vi "Read SS2 DAQ Parameters.vi"(8 "error in (no error)":errorcluster, 11 "group in":T3 format="%.0x") -> (0 "error out":errorcluster, 1 "FPGA Parameters":T1 {"gs_psincdec 3" format="%0.0f"; "gs_psincdec 2" format="%0.0f"; "gs_psincdec_1" format="%0.0f"; "gs_no_shift_adj_3" format="%0.0f"; "gs_no_shift_adj_2" format="%0.0f"; "gs_psincdec_0" format="%0.0f"}, 2 "DAQ Parameters":T2 {"# Gate Positions" format="%0.0f"; "Gate Offset" format="%0.0f"; "Bitness" format="%0.0f"; "# Gate Set" format="%0.0f"}, 3 "group out":T3 format="%.0x")   [LabVIEW 2021, in "SwissSPAD.lvlib"]
uses:
  SwissSPAD.lvlib
  <vilib>/addons/h5labview2/base/hid_t.ctl
  SS2 DAQ Parameters.ctl
  SS2 FPGA Parameters.ctl
  SS2 DAQ Parameters List.ctl
  <vilib>/addons/h5labview2/base/lib_path.vi
  <vilib>/addons/h5labview2/base/H5Equery.vi
  <vilib>/addons/h5labview2/dataset/H5Dread.llb/H5Dread.xnode
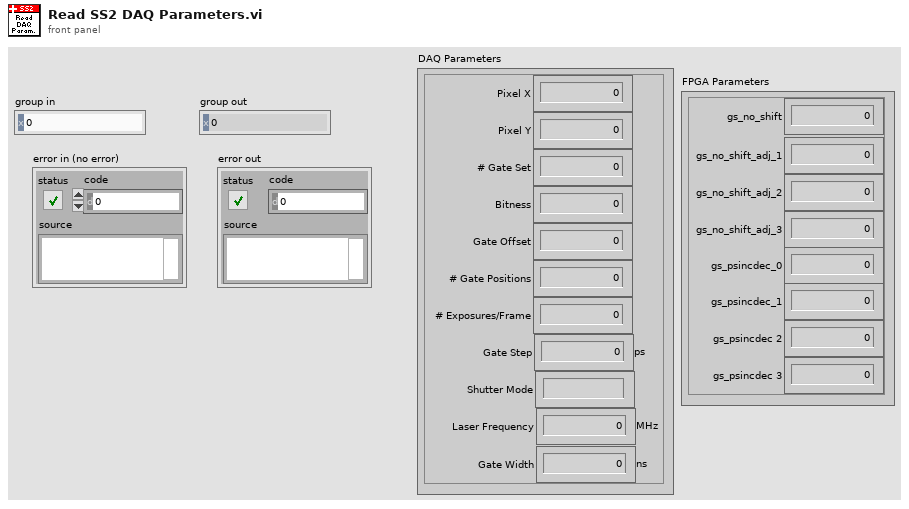
[diagram p1: front panel]
types:
  T1 = typedef "SwissSPAD.lvlib/SS2 FPGA Parameters.ctl" = cluster{"gs_no_shift":i32, "gs_no_shift_adj_1":u32, "gs_no_shift_adj_2":u32, "gs_no_shift_adj_3":u32, "gs_psincdec_0":i32, "gs_psincdec_1":u32, "gs_psincdec 2":u32, "gs_psincdec 3":u32}
  T2 = typedef "SwissSPAD.lvlib/SS2 DAQ Parameters.ctl" = cluster{"Pixel X":i32, "Pixel Y":i32, "# Gate Set":i32, "Bitness":i32, "Gate Offset":i32, "# Gate Positions":i32, "# Exposures/Frame ":i32, "Gate Step":dbl[unit], "Shutter Mode":string, "Laser Frequency":dbl[unit], "Gate Width":dbl[unit]}
  T3 = typedef "hid_t.ctl" = i64
  T4 = typedef "SwissSPAD.lvlib/SS2 DAQ Parameters List.ctl" = enum16{"---DAQ Parameters---", "bits_10", "exp_no_seq", "gate_offset", "gate_set_no", "gate_step_ps", "gs_no_shift", "no_gate_pos", "pixel_x", "pixel_y", "shutter_mode", "gate_width_ns", "laser_f_MHz", "---FPGA Parameters---", "gs_no_shift_adj_1", "gs_no_shift_adj_2", "gs_no_shift_adj_3", "gs_psincdec_0", "gs_psincdec_1", "gs_psincdec_2", "gs_psincdec_3"}
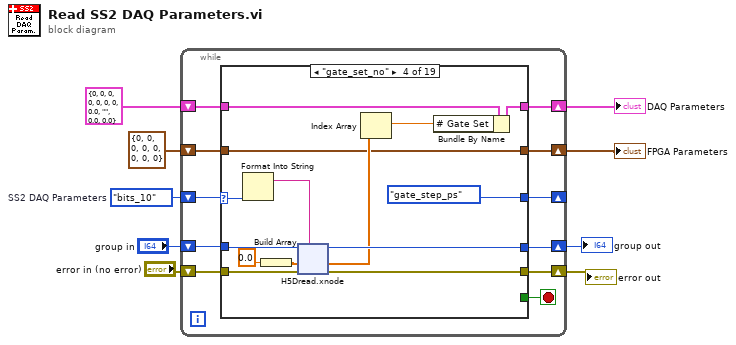
[diagram p0: block diagram]
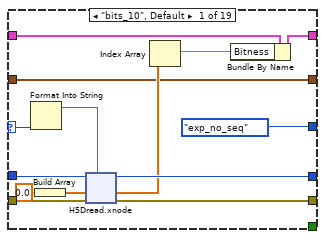
[diagram p2: hidden frame]
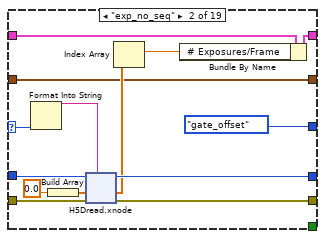
[diagram p3: hidden frame]
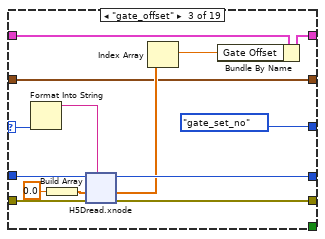
[diagram p4: hidden frame]
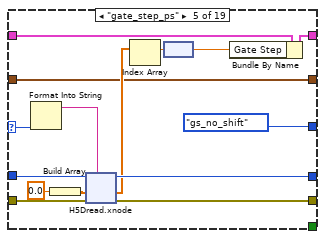
[diagram p5: hidden frame]
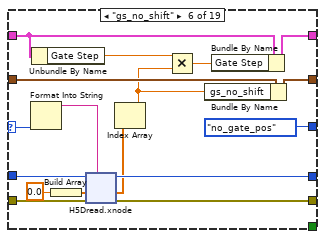
[diagram p6: hidden frame]
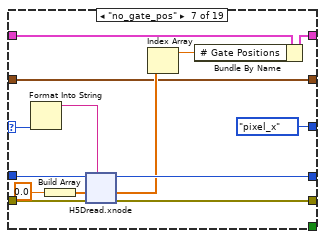
[diagram p7: hidden frame]
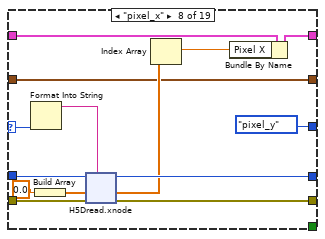
[diagram p8: hidden frame]
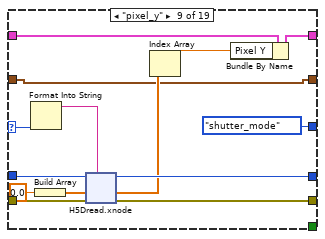
[diagram p9: hidden frame]
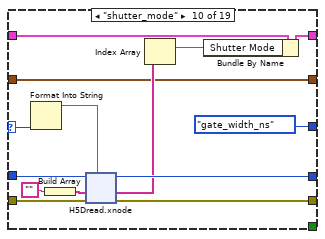
[diagram p10: hidden frame]
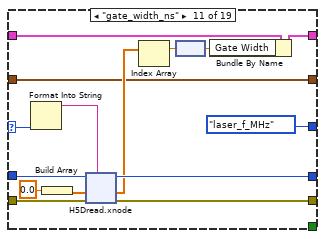
[diagram p11: hidden frame]
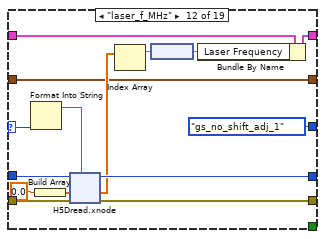
[diagram p12: hidden frame]
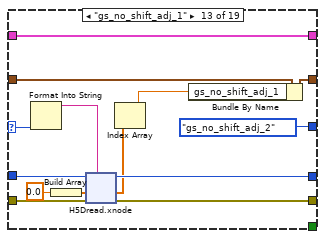
[diagram p13: hidden frame]
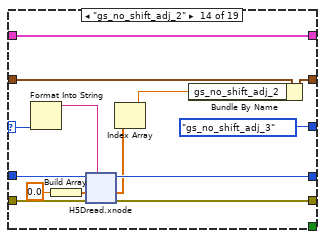
[diagram p14: hidden frame]
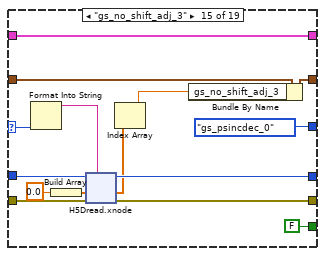
[diagram p15: hidden frame]
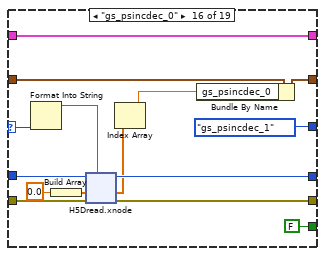
[diagram p16: hidden frame]
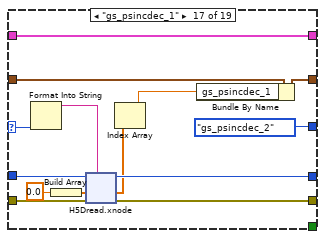
[diagram p17: hidden frame]
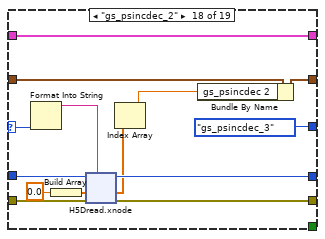
[diagram p18: hidden frame]
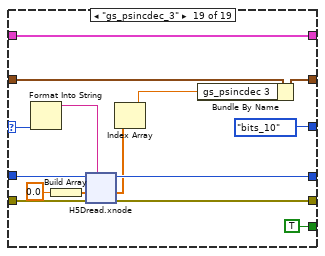
[diagram p19: hidden frame]
diagram:
  w5 = SS2_DAQ_Parameters_List."bits_10"  # SS2 DAQ Parameters
  n1 = while {
    shift-right: [w14] -> w8
    shift-left: T2 {"Pixel X"=0, "Pixel Y"=0, "# Gate Set"=0, "Bitness"=0, "Gate Offset"=0, "# Gate Positions"=0, "# Exposures/Frame "=0, "Gate Step"=0.0, "Shutter Mode"="", "Laser Frequency"=0.0, "Gate Width"=0.0} ("DAQ Parameters") -> [w15]
    shift-right: [w16] -> w6
    shift-left: "error in (no error)" -> [w17]
    shift-right: [w18] -> w3
    shift-left: "group in" -> [w19]
    shift-right: [w12] -> _
    shift-left: w5 -> [w20]
    shift-right: [w10] -> w1
    shift-left: T1 {"gs_no_shift"=0, "gs_no_shift_adj_1"=0, "gs_no_shift_adj_2"=0, "gs_no_shift_adj_3"=0, "gs_psincdec_0"=0, "gs_psincdec_1"=0, "gs_psincdec 2"=0, "gs_psincdec 3"=0} ("FPGA Parameters") -> [w11]
    stop <- w13 stop-if-true
    n2 = case shown="\"gate_set_no\"" w20 {
      selector: w20 -> [w33 w62 w91 w120 w150 w182 w211 w240 w269 w298 w328 w358 w387 w416 w446 w476 w505 w534 w564]
      tunnel: w19 -> [w32 w61 w90 w119 w149 w181 w210 w239 w268 w297 w327 w357 w386 w415 w445 w475 w504 w533 w563]
      tunnel: [w31 w60 w89 w118 w148 w180 w209 w238 w267 w296 w326 w356 w385 w414 w444 w474 w503 w532 w562] -> w18
      tunnel: w17 -> [w30 w59 w88 w117 w147 w179 w208 w237 w266 w295 w325 w355 w384 w413 w443 w473 w502 w531 w561]
      tunnel: [w29 w58 w87 w116 w146 w178 w207 w236 w265 w294 w324 w354 w383 w412 w442 w472 w501 w530 w560] -> w16
      tunnel: w15 -> [w27 w56 w85 w114 w144 w170 w205 w234 w263 w292 w323 w352 w377 w406 w436 w466 w495 w524 w554]
      tunnel: [w25 w54 w83 w112 w142 w171 w203 w232 w261 w290 w321 w350 w377 w406 w436 w466 w495 w524 w554] -> w14
      tunnel: [_ _ _ _ _ _ _ _ _ _ _ _ _ _ FALSE FALSE _ _ TRUE] -> w13
      tunnel: [SS2_DAQ_Parameters_List."exp_no_seq" ("SS2 DAQ Parameters") SS2_DAQ_Parameters_List."gate_offset" ("SS2 DAQ Parameters") SS2_DAQ_Parameters_List."gate_set_no" ("SS2 DAQ Parameters") SS2_DAQ_Parameters_List."gate_step_ps" ("SS2 DAQ Parameters") SS2_DAQ_Parameters_List."gs_no_shift" ("SS2 DAQ Parameters") SS2_DAQ_Parameters_List."no_gate_pos" ("SS2 DAQ Parameters") SS2_DAQ_Parameters_List."pixel_x" ("SS2 DAQ Parameters") SS2_DAQ_Parameters_List."pixel_y" ("SS2 DAQ Parameters") SS2_DAQ_Parameters_List."shutter_mode" ("SS2 DAQ Parameters") SS2_DAQ_Parameters_List."gate_width_ns" ("SS2 DAQ Parameters") SS2_DAQ_Parameters_List."laser_f_MHz" ("SS2 DAQ Parameters") SS2_DAQ_Parameters_List."gs_no_shift_adj_1" ("SS2 DAQ Parameters") SS2_DAQ_Parameters_List."gs_no_shift_adj_2" ("SS2 DAQ Parameters") SS2_DAQ_Parameters_List."gs_no_shift_adj_3" ("SS2 DAQ Parameters") SS2_DAQ_Parameters_List."gs_psincdec_0" ("SS2 DAQ Parameters") SS2_DAQ_Parameters_List."gs_psincdec_1" ("SS2 DAQ Parameters") SS2_DAQ_Parameters_List."gs_psincdec_2" ("SS2 DAQ Parameters") SS2_DAQ_Parameters_List."gs_psincdec_3" ("SS2 DAQ Parameters") SS2_DAQ_Parameters_List."bits_10" ("SS2 DAQ Parameters")] -> w12
      tunnel: w11 -> [w21 w50 w79 w108 w137 w173 w199 w228 w257 w286 w318 w345 w376 w405 w435 w465 w494 w523 w553]
      tunnel: [w21 w50 w79 w108 w137 w172 w199 w228 w257 w286 w318 w345 w375 w404 w434 w464 w493 w522 w552] -> w10
      frame "bits_10", Default {
        n3 = Format Into String(w33) -> (resulting string=w34:string)  [unwired: 3 in, 1 out]
        n4 = Build Array(0.0) -> (w24:dbl[])
        n5 = xnode "H5Dread.xnode"("dataset name (this)"=w34, "error in (no error)"=w30, "default"=w24, "ref in"=w32) -> ("error out"=w29:errorcluster, "data"=w26:dbl[], "ref out"=w31:T3)  [unwired: 2 in, 1 out]
        n6 = Index Array(array=w26) -> (element=w23:dbl)  [unwired: 1 in]
        n7 = Bundle By Name(cluster=w27, "Bitness"=w23) -> (w25:T2)
      }
      frame "exp_no_seq" {
        n8 = Format Into String(w62) -> (resulting string=w63:string)  [unwired: 3 in, 1 out]
        n9 = Build Array(0.0) -> (w53:dbl[])
        n10 = xnode "H5Dread.xnode"("dataset name (this)"=w63, "error in (no error)"=w59, "default"=w53, "ref in"=w61) -> ("error out"=w58:errorcluster, "data"=w55:dbl[], "ref out"=w60:T3)  [unwired: 2 in, 1 out]
        n11 = Index Array(array=w55) -> (element=w52:dbl)  [unwired: 1 in]
        n12 = Bundle By Name(cluster=w56, "# Exposures/Frame"=w52) -> (w54:T2)
      }
      frame "gate_offset" {
        n13 = Format Into String(w91) -> (resulting string=w92:string)  [unwired: 3 in, 1 out]
        n14 = Build Array(0.0) -> (w82:dbl[])
        n15 = xnode "H5Dread.xnode"("dataset name (this)"=w92, "error in (no error)"=w88, "default"=w82, "ref in"=w90) -> ("error out"=w87:errorcluster, "data"=w84:dbl[], "ref out"=w89:T3)  [unwired: 2 in, 1 out]
        n16 = Index Array(array=w84) -> (element=w81:dbl)  [unwired: 1 in]
        n17 = Bundle By Name(cluster=w85, "Gate Offset"=w81) -> (w83:T2)
      }
      frame "gate_set_no" {
        n18 = Format Into String(w120) -> (resulting string=w121:string)  [unwired: 3 in, 1 out]
        n19 = Build Array(0.0) -> (w111:dbl[])
        n20 = xnode "H5Dread.xnode"("dataset name (this)"=w121, "error in (no error)"=w117, "default"=w111, "ref in"=w119) -> ("error out"=w116:errorcluster, "data"=w113:dbl[], "ref out"=w118:T3)  [unwired: 2 in, 1 out]
        n21 = Index Array(array=w113) -> (element=w110:dbl)  [unwired: 1 in]
        n22 = Bundle By Name(cluster=w114, "# Gate Set"=w110) -> (w112:T2)
      }
      frame "gate_step_ps" {
        n23 = Format Into String(w150) -> (resulting string=w151:string)  [unwired: 3 in, 1 out]
        n24 = Build Array(0.0) -> (w141:dbl[])
        n25 = xnode "H5Dread.xnode"("dataset name (this)"=w151, "error in (no error)"=w147, "default"=w141, "ref in"=w149) -> ("error out"=w146:errorcluster, "data"=w143:dbl[], "ref out"=w148:T3)  [unwired: 2 in, 1 out]
        n26 = Index Array(array=w143) -> (element=w140:dbl)  [unwired: 1 in]
        n27 = node(w140) -> (w138:dbl[unit])
        n28 = Bundle By Name(cluster=w144, "Gate Step"=w138) -> (w142:T2)
      }
      frame "gs_no_shift" {
        n29 = Format Into String(w182) -> (resulting string=w183:string)  [unwired: 3 in, 1 out]
        n30 = Unbundle By Name(w170) -> ("Gate Step"=w169:dbl[unit])
        n31 = Build Array(0.0) -> (w175:dbl[])
        n32 = xnode "H5Dread.xnode"("dataset name (this)"=w183, "error in (no error)"=w179, "default"=w175, "ref in"=w181) -> ("error out"=w178:errorcluster, "data"=w176:dbl[], "ref out"=w180:T3)  [unwired: 2 in, 1 out]
        n33 = Index Array(array=w176) -> (element=w168:dbl)  [unwired: 1 in]
        n34 = Multiply(x=w169, y=w168) -> (x*y=w167:dbl[unit])
        n35 = Bundle By Name(cluster=w173, "gs_no_shift"=w168) -> (w172:T1)
        n36 = Bundle By Name(cluster=w170, "Gate Step"=w167) -> (w171:T2)
      }
      frame "no_gate_pos" {
        n37 = Format Into String(w211) -> (resulting string=w212:string)  [unwired: 3 in, 1 out]
        n38 = Build Array(0.0) -> (w202:dbl[])
        n39 = xnode "H5Dread.xnode"("dataset name (this)"=w212, "error in (no error)"=w208, "default"=w202, "ref in"=w210) -> ("error out"=w207:errorcluster, "data"=w204:dbl[], "ref out"=w209:T3)  [unwired: 2 in, 1 out]
        n40 = Index Array(array=w204) -> (element=w201:dbl)  [unwired: 1 in]
        n41 = Bundle By Name(cluster=w205, "# Gate Positions"=w201) -> (w203:T2)
      }
      frame "pixel_x" {
        n42 = Format Into String(w240) -> (resulting string=w241:string)  [unwired: 3 in, 1 out]
        n43 = Build Array(0.0) -> (w231:dbl[])
        n44 = xnode "H5Dread.xnode"("dataset name (this)"=w241, "error in (no error)"=w237, "default"=w231, "ref in"=w239) -> ("error out"=w236:errorcluster, "data"=w233:dbl[], "ref out"=w238:T3)  [unwired: 2 in, 1 out]
        n45 = Index Array(array=w233) -> (element=w230:dbl)  [unwired: 1 in]
        n46 = Bundle By Name(cluster=w234, "Pixel X"=w230) -> (w232:T2)
      }
      frame "pixel_y" {
        n47 = Format Into String(w269) -> (resulting string=w270:string)  [unwired: 3 in, 1 out]
        n48 = Build Array(0.0) -> (w260:dbl[])
        n49 = xnode "H5Dread.xnode"("dataset name (this)"=w270, "error in (no error)"=w266, "default"=w260, "ref in"=w268) -> ("error out"=w265:errorcluster, "data"=w262:dbl[], "ref out"=w267:T3)  [unwired: 2 in, 1 out]
        n50 = Index Array(array=w262) -> (element=w259:dbl)  [unwired: 1 in]
        n51 = Bundle By Name(cluster=w263, "Pixel Y"=w259) -> (w261:T2)
      }
      frame "shutter_mode" {
        n52 = Format Into String(w298) -> (resulting string=w299:string)  [unwired: 3 in, 1 out]
        n53 = Build Array("") -> (w289:string[])
        n54 = xnode "H5Dread.xnode"("dataset name (this)"=w299, "error in (no error)"=w295, "default"=w289, "ref in"=w297) -> ("error out"=w294:errorcluster, "data"=w291:string[], "ref out"=w296:T3)  [unwired: 2 in, 1 out]
        n55 = Index Array(array=w291) -> (element=w288:string)  [unwired: 1 in]
        n56 = Bundle By Name(cluster=w292, "Shutter Mode"=w288) -> (w290:T2)
      }
      frame "gate_width_ns" {
        n57 = Format Into String(w328) -> (resulting string=w329:string)  [unwired: 3 in, 1 out]
        n58 = Build Array(0.0) -> (w316:dbl[])
        n59 = xnode "H5Dread.xnode"("dataset name (this)"=w329, "error in (no error)"=w325, "default"=w316, "ref in"=w327) -> ("error out"=w324:errorcluster, "data"=w322:dbl[], "ref out"=w326:T3)  [unwired: 2 in, 1 out]
        n60 = Index Array(array=w322) -> (element=w320:dbl)  [unwired: 1 in]
        n61 = node(w320) -> (w315:dbl[unit])
        n62 = Bundle By Name(cluster=w323, "Gate Width"=w315) -> (w321:T2)
      }
      frame "laser_f_MHz" {
        n63 = Format Into String(w358) -> (resulting string=w359:string)  [unwired: 3 in, 1 out]
        n64 = Build Array(0.0) -> (w349:dbl[])
        n65 = xnode "H5Dread.xnode"("dataset name (this)"=w359, "error in (no error)"=w355, "default"=w349, "ref in"=w357) -> ("error out"=w354:errorcluster, "data"=w351:dbl[], "ref out"=w356:T3)  [unwired: 2 in, 1 out]
        n66 = Index Array(array=w351) -> (element=w348:dbl)  [unwired: 1 in]
        n67 = node(w348) -> (w346:dbl[unit])
        n68 = Bundle By Name(cluster=w352, "Laser Frequency"=w346) -> (w350:T2)
      }
      frame "gs_no_shift_adj_1" {
        n69 = Format Into String(w387) -> (resulting string=w388:string)  [unwired: 3 in, 1 out]
        n70 = Build Array(0.0) -> (w380:dbl[])
        n71 = xnode "H5Dread.xnode"("dataset name (this)"=w388, "error in (no error)"=w384, "default"=w380, "ref in"=w386) -> ("error out"=w383:errorcluster, "data"=w381:dbl[], "ref out"=w385:T3)  [unwired: 2 in, 1 out]
        n72 = Index Array(array=w381) -> (element=w379:dbl)  [unwired: 1 in]
        n73 = Bundle By Name(cluster=w376, "gs_no_shift_adj_1"=w379) -> (w375:T1)
      }
      frame "gs_no_shift_adj_2" {
        n74 = Format Into String(w416) -> (resulting string=w417:string)  [unwired: 3 in, 1 out]
        n75 = Build Array(0.0) -> (w409:dbl[])
        n76 = xnode "H5Dread.xnode"("dataset name (this)"=w417, "error in (no error)"=w413, "default"=w409, "ref in"=w415) -> ("error out"=w412:errorcluster, "data"=w410:dbl[], "ref out"=w414:T3)  [unwired: 2 in, 1 out]
        n77 = Index Array(array=w410) -> (element=w408:dbl)  [unwired: 1 in]
        n78 = Bundle By Name(cluster=w405, "gs_no_shift_adj_2"=w408) -> (w404:T1)
      }
      frame "gs_no_shift_adj_3" {
        n79 = Format Into String(w446) -> (resulting string=w447:string)  [unwired: 3 in, 1 out]
        n80 = Build Array(0.0) -> (w439:dbl[])
        n81 = xnode "H5Dread.xnode"("dataset name (this)"=w447, "error in (no error)"=w443, "default"=w439, "ref in"=w445) -> ("error out"=w442:errorcluster, "data"=w440:dbl[], "ref out"=w444:T3)  [unwired: 2 in, 1 out]
        n82 = Index Array(array=w440) -> (element=w438:dbl)  [unwired: 1 in]
        n83 = Bundle By Name(cluster=w435, "gs_no_shift_adj_3"=w438) -> (w434:T1)
      }
      frame "gs_psincdec_0" {
        n84 = Format Into String(w476) -> (resulting string=w477:string)  [unwired: 3 in, 1 out]
        n85 = Build Array(0.0) -> (w469:dbl[])
        n86 = xnode "H5Dread.xnode"("dataset name (this)"=w477, "error in (no error)"=w473, "default"=w469, "ref in"=w475) -> ("error out"=w472:errorcluster, "data"=w470:dbl[], "ref out"=w474:T3)  [unwired: 2 in, 1 out]
        n87 = Index Array(array=w470) -> (element=w468:dbl)  [unwired: 1 in]
        n88 = Bundle By Name(cluster=w465, "gs_psincdec_0"=w468) -> (w464:T1)
      }
      frame "gs_psincdec_1" {
        n89 = Format Into String(w505) -> (resulting string=w506:string)  [unwired: 3 in, 1 out]
        n90 = Build Array(0.0) -> (w498:dbl[])
        n91 = xnode "H5Dread.xnode"("dataset name (this)"=w506, "error in (no error)"=w502, "default"=w498, "ref in"=w504) -> ("error out"=w501:errorcluster, "data"=w499:dbl[], "ref out"=w503:T3)  [unwired: 2 in, 1 out]
        n92 = Index Array(array=w499) -> (element=w497:dbl)  [unwired: 1 in]
        n93 = Bundle By Name(cluster=w494, "gs_psincdec_1"=w497) -> (w493:T1)
      }
      frame "gs_psincdec_2" {
        n94 = Format Into String(w534) -> (resulting string=w535:string)  [unwired: 3 in, 1 out]
        n95 = Build Array(0.0) -> (w527:dbl[])
        n96 = xnode "H5Dread.xnode"("dataset name (this)"=w535, "error in (no error)"=w531, "default"=w527, "ref in"=w533) -> ("error out"=w530:errorcluster, "data"=w528:dbl[], "ref out"=w532:T3)  [unwired: 2 in, 1 out]
        n97 = Index Array(array=w528) -> (element=w526:dbl)  [unwired: 1 in]
        n98 = Bundle By Name(cluster=w523, "gs_psincdec 2"=w526) -> (w522:T1)
      }
      frame "gs_psincdec_3" {
        n99 = Format Into String(w564) -> (resulting string=w565:string)  [unwired: 3 in, 1 out]
        n100 = Build Array(0.0) -> (w557:dbl[])
        n101 = xnode "H5Dread.xnode"("dataset name (this)"=w565, "error in (no error)"=w561, "default"=w557, "ref in"=w563) -> ("error out"=w560:errorcluster, "data"=w558:dbl[], "ref out"=w562:T3)  [unwired: 2 in, 1 out]
        n102 = Index Array(array=w558) -> (element=w556:dbl)  [unwired: 1 in]
        n103 = Bundle By Name(cluster=w553, "gs_psincdec 3"=w556) -> (w552:T1)
      }
    }
  }
  "group out" <- w3
  "error out" <- w6
  "DAQ Parameters" <- w8
  "FPGA Parameters" <- w1
